vi "Make DeltaJSON Subs.vi"(6 "Array":T1(array[cluster]), 8 "delta":cluster{"token type":T2, "Type Definition":T3}[](array[cluster]), 9 "Delta JSON":string, 10 "orig":cluster{"token type":T2, "Type Definition":T3}[](array[cluster]), 11 "orig string":string) -> (3 "result string":string)   [LabVIEW 2019]
uses:
  <vilib>/MultiError/TokenizeJSON/JSON Token Values.ctl
  <vilib>/MultiError/Errors Cluster Multiple Errors/JSON Token Descriptor.ctl
  <vilib>/MultiError/TokenizeJSON/JSON Raw Token Values.ctl
  <vilib>/MultiError/TokenizeJSON/Multi Error Cluster.lvlib
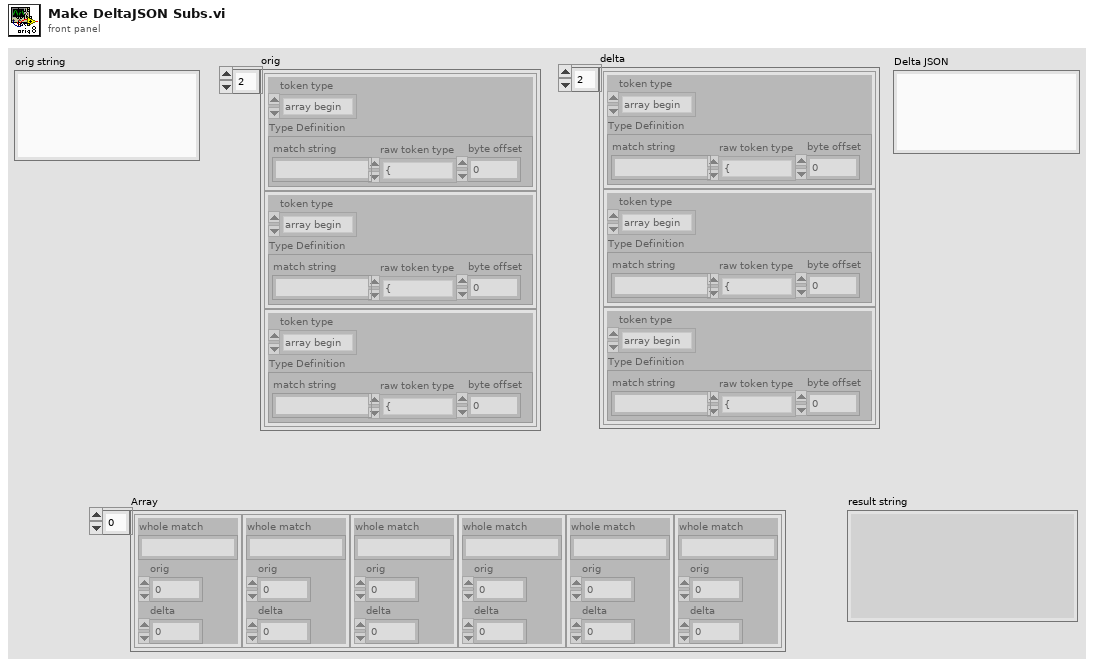
[diagram p1: front panel]
types:
  T1 = cluster{"whole match":string, "orig":i32, "delta":i32}[]
  T2 = typedef "Multi Error Cluster.lvlib/JSON Token Values.ctl" = enum32{"array begin", "array end", "object begin", "object end", "value", "invalid", "name"}
  T3 = typedef "Multi Error Cluster.lvlib/JSON Token Descriptor.ctl" = cluster{"match string":string, "raw token type":T4, "byte offset ":i32}
  T4 = typedef "Multi Error Cluster.lvlib/JSON Raw Token Values.ctl" = enum32{"{", "}", "[", "]", ",", ":", "\"", "number", "string", "true", "false", "null", "invalid"}
  T5 = cluster{"whole match":string, "orig":i32, "delta":i32}
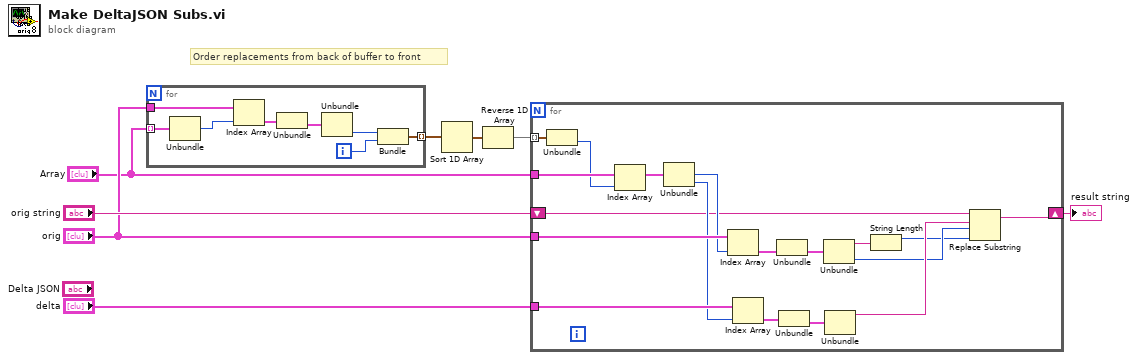
[diagram p0: block diagram]
diagram:
  # "Order replacements from back of buffer to front"
  n1 = for {
    tunnel: "Array" -> [w16] mode=indexing
    tunnel: "orig" -> [w15]
    tunnel: [w9] -> w4 mode=indexing
    i -> [w10]
    n2 = Unbundle(w16) -> ("orig"=w14:i32)  [unwired: 2 out]
    n3 = Index Array(array=w15, index=w14) -> (element=w13:cluster{"token type":T2, "Type Definition":T3})
    n4 = Unbundle(w13) -> ("Type Definition"=w12:T3)  [unwired: 1 out]
    n5 = Unbundle(w12) -> ("byte offset"=w11:i32)  [unwired: 2 out]
    n6 = Bundle("byte offset"=w11, w10) -> (w9:cluster{"byte offset ":i32, i32})  [unwired: 1 in]
  }
  n7 = Sort 1D Array(array=w4) -> (sorted array=w3:cluster{"byte offset ":i32, i32}[])
  n8 = Reverse 1D Array(array=w3) -> (reversed array=w2:cluster{"byte offset ":i32, i32}[])
  n9 = for {
    tunnel: "Array" -> [w20]
    tunnel: "orig" -> [w34]
    tunnel: "delta" -> [w33]
    tunnel: w2 -> [w21] mode=indexing
    shift-right: [w17] -> w1
    shift-left: "orig string" -> [w26]
    n10 = Unbundle(w21) -> (w19:i32)  [unwired: 1 out]
    n11 = Index Array(array=w20, index=w19) -> (element=w18:T5)
    n12 = Unbundle(w18) -> ("orig"=w32:i32, "delta"=w31:i32)  [unwired: 1 out]
    n13 = Index Array(array=w34, index=w32) -> (element=w30:cluster{"token type":T2, "Type Definition":T3})
    n14 = Index Array(array=w33, index=w31) -> (element=w29:cluster{"token type":T2, "Type Definition":T3})
    n15 = Unbundle(w30) -> ("Type Definition"=w27:T3)  [unwired: 1 out]
    n16 = Unbundle(w29) -> ("Type Definition"=w28:T3)  [unwired: 1 out]
    n17 = Unbundle(w27) -> ("match string"=w23:string, "byte offset"=w24:i32)  [unwired: 1 out]
    n18 = Unbundle(w28) -> ("match string"=w25:string)  [unwired: 2 out]
    n19 = String Length(string=w23) -> (length=w22:i32)
    n20 = Replace Substring(2:w22, 3:w24, 4:w25, 5:w26) -> (1:w17:string)  [unwired: 1 out]
  }
  "result string" <- w1
